vi "DT_Pre_Scale.vi"(11 "Points In":cluster{"x":dbl, "y":dbl, "index":i32}[](array[cluster])) -> (2 "scale factor":dbl, 3 "Points Out":cluster{"x":dbl, "y":dbl, "index":i32}[](array[cluster]))   [LabVIEW 2020, in "NI_AAL_Geometry.lvlib"]
uses:
  <vilib>/Analysis/NI_AAL_Geometry.lvlib
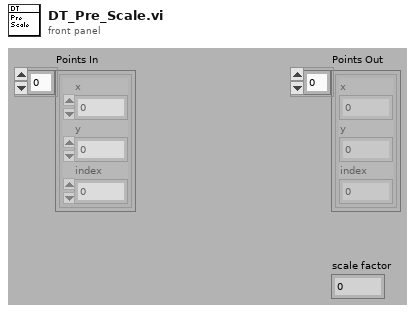
[diagram p1: front panel]
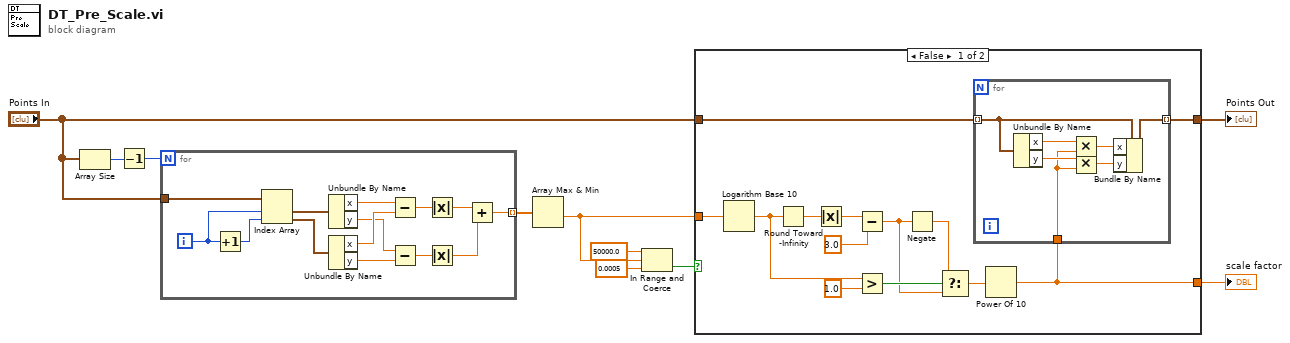
[diagram p0: block diagram]
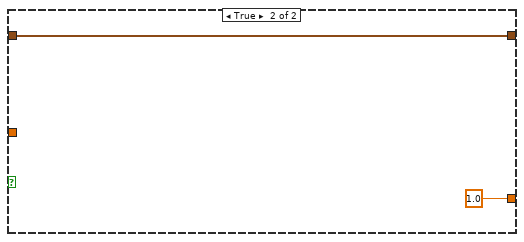
[diagram p2: hidden frame]
diagram:
  n1 = Array Size(array="Points In") -> (size(s)=w10:i32)
  n2 = Decrement(x=w10) -> (x-1=w9:i32)
  n3 = for {
    N: w9 -> [_]
    tunnel: "Points In" -> [w24]
    tunnel: [w11] -> w8 mode=indexing
    i -> [w22]
    n4 = Increment(x=w22) -> (x+1=w23:i32)
    n5 = Index Array(array=w24, index #1=w22, index #2=w23) -> (element #1=w21:cluster{"x":dbl, "y":dbl, "index":i32}, element #2=w20:cluster{"x":dbl, "y":dbl, "index":i32})
    n6 = Unbundle By Name(w21) -> ("x"=w19:dbl, "y"=w17:dbl)
    n7 = Unbundle By Name(w20) -> ("x"=w18:dbl, "y"=w16:dbl)
    n8 = Subtract(x=w19, y=w18) -> (x-y=w15:dbl)
    n9 = Subtract(x=w17, y=w16) -> (x-y=w14:dbl)
    n10 = Absolute Value(x=w15) -> (abs(x)=w13:dbl)
    n11 = Absolute Value(x=w14) -> (abs(x)=w12:dbl)
    n12 = Add(x=w13, y=w12) -> (x+y=w11:dbl)
  }
  n13 = Array Max & Min(array=w8) -> (min value=w4:dbl)  [unwired: 3 out]
  n14 = In Range and Coerce(upper limit=50000.0, x=w4, lower limit=0.0005) -> (In Range?=w5:bool)  [unwired: 1 out]
  n15 = case shown="False" w5 {
    tunnel: w4 -> [w29 _]
    tunnel: "Points In" -> [w28 w46]
    tunnel: [w27 w46] -> w2
    tunnel: [w25 1.0] -> w3
    frame False {
      n16 = Logarithm Base 10(1:w29) -> (0:w33:dbl)
      n17 = Round Toward -Infinity(1:w33) -> (0:w30:dbl)
      n18 = Absolute Value(x=w30) -> (abs(x)=w31:dbl)
      n19 = Subtract(x=w31, y=3.0) -> (x-y=w26:dbl)
      n20 = Greater?(x=w33, y=1.0) -> (0:w35:bool)
      n21 = Negate(x=w26) -> (-x=w36:dbl)
      n22 = Select(t=w36, s=w35, f=w26) -> (s? t:f=w37:dbl)
      n23 = Power Of 10(x=w37) -> (10^x=w25:dbl)
      n24 = for {
        tunnel: w28 -> [w44] mode=indexing
        tunnel: w25 -> [w41]
        tunnel: [w38] -> w27 mode=indexing
        n25 = Unbundle By Name(w44) -> ("x"=w43:dbl, "y"=w42:dbl)
        n26 = Multiply(x=w43, y=w41) -> (x*y=w40:dbl)
        n27 = Multiply(x=w42, y=w41) -> (x*y=w39:dbl)
        n28 = Bundle By Name(cluster=w44, "x"=w40, "y"=w39) -> (w38:cluster{"x":dbl, "y":dbl, "index":i32})
      }
    }
    frame True {
    }
  }
  "Points Out" <- w2
  "scale factor" <- w3
